vi "csv_separador_sub.vi"(5 "Archivo de referencias (.csv)":path) -> (0 "subarray 2":string[][](array[string]), 1 "subarray":string[][](array[string]), 2 "all rows":string[][](array[string]))   [LabVIEW 2017]
uses:
  <vilib>/Utility/file.llb/Read Delimited Spreadsheet (string).vi
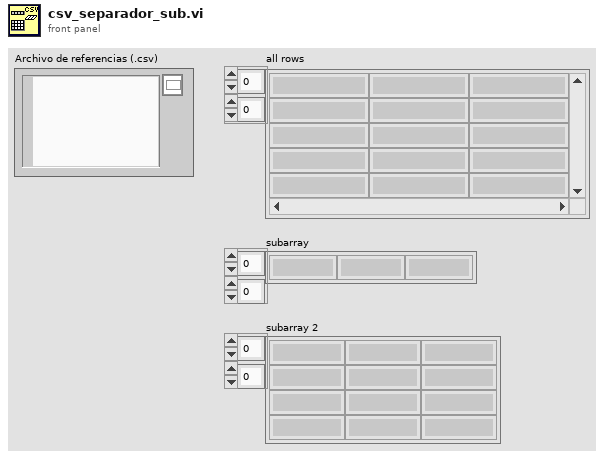
[diagram p1: front panel]
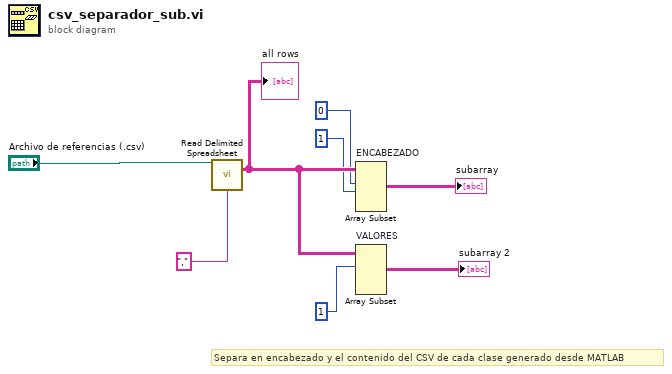
[diagram p0: block diagram]
diagram:
  # "Separa en encabezado y el contenido del CSV de cada clase generado desde MATLAB"
  n1 = call-poly <vilib>:"Read Delimited Spreadsheet.vi"("file path (dialog if empty)"="Archivo de referencias (.csv)", "delimiter (\\t)"="," ("delimiter (\\t)")) -> ("all rows"=w7:string[][])  [unwired: 8 in, 5 out]
  "all rows" <- w7
  n2 = Array Subset "ENCABEZADO"(array=w7, index (row)=0 ("index"), length (row)=1 ("length")) -> (→"subarray":string[][])  [unwired: 2 in]
  n3 = Array Subset "VALORES"(array=w7, index (row)=1 ("index")) -> (→"subarray 2":string[][])  [unwired: 3 in]
